vi "CaseVsEvent.vi"() -> ()   [LabVIEW 2012]
panel:
  in  "Button3 (switch)":bool
  in  "Button2 (latch)":bool
  in  "Button1 (latch)":bool
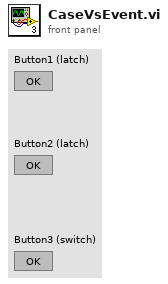
[diagram p1: front panel]
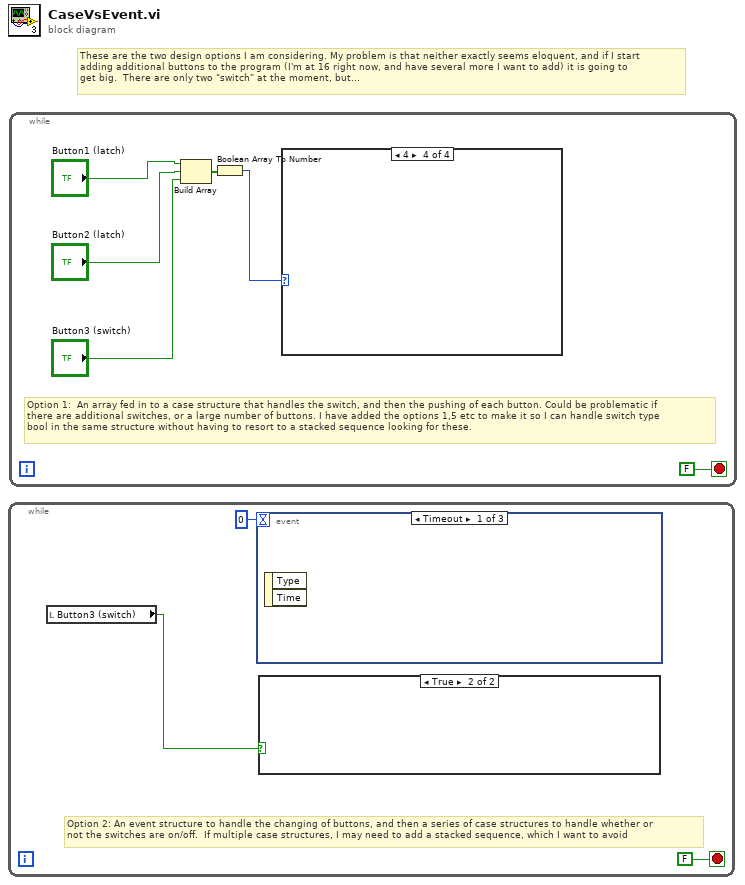
[diagram p0: block diagram]
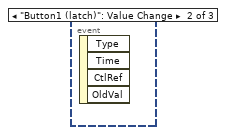
[diagram p2: hidden frame]
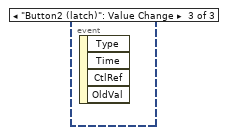
[diagram p3: hidden frame]
diagram:
  # "These are the two design options I am considering. My problem is that neither exactly seems eloquent, and if I start\nadding additional buttons to the program (I'm at 16 right now, and have several more I want to add) it is going to\nget big.  There are only two \"switch\" at the moment, but..."
  n1 = while {
    stop <- FALSE stop-if-true
    # "Option 2: An event structure to handle the changing of buttons, and then a series of case structures to handle whether or\nnot the switches are on/off.  If multiple case structures, I may need to add a stacked sequence, which I want to avoid"
    n2 = local read "Button3 (switch)"() -> (w3:bool)
    n3 = event shown="[0] Timeout" {
      selector: _ -> [_ _ _]
      dyn-events: _ -> [_ _ _]
      timeout: 0 -> [_ _ _]
      event Timeout {
        n4 = event-data() -> ()  [unwired: 1 in, 2 out]
      }
      event "Button1 (latch)": Value Change {
        n5 = event-data() -> ()  [unwired: 1 in, 4 out]
      }
      event "Button2 (latch)": Value Change {
        n6 = event-data() -> ()  [unwired: 1 in, 4 out]
      }
    }
    n7 = case shown="True" w3 {
      frame False {
      }
      frame True {
      }
    }
  }
  n8 = while {
    stop <- FALSE stop-if-true
    # "Option 1:  An array fed in to a case structure that handles the switch, and then the pushing of each button. Could be problematic if\nthere are additional switches, or a large number of buttons. I have added the options 1,5 etc to make it so I can handle switch type\nbool in the same structure without having to resort to a stacked sequence looking for these."
    n9 = Build Array("Button1 (latch)", "Button2 (latch)", "Button3 (switch)") -> (w9:bool[])
    n10 = Boolean Array To Number(Boolean array=w9) -> (number=w8:u32)
    n11 = case shown="4" w8 {
      frame 0, Default {
      }
      frame 1, 5 {
      }
      frame 2, 6 {
      }
      frame 4 {
      }
    }
  }
